vi "getConstants.vi"(0 "niDAQmxAO.lvclass in":refnum<class "niDAQmxAO.lvclass">, 1 "error in (no error)":errorcluster) -> (2 "niDAQmxAO.lvclass out":refnum<class "niDAQmxAO.lvclass">, 3 "Constants":T1={"Configuration Type"={"Differential"=10106, "Pseudodifferential"=12529, "RSE"=10083.0}, "Voltage Type"={"Voltage"="Voltage", "Current"="Current", "Standard Function "={"Sine"="Sine", "Square"="Square", "Triangle"="Triangle"}}}, 4 "error out":errorcluster)   [LabVIEW 2011, in "Hardware.lvlib" / "Channels.lvlib" / "niDAQmxAO.lvclass"]
uses:
  niDAQmxAO.lvclass
  niDAQmxAO.lvclass/niDAQmxAO.ctl
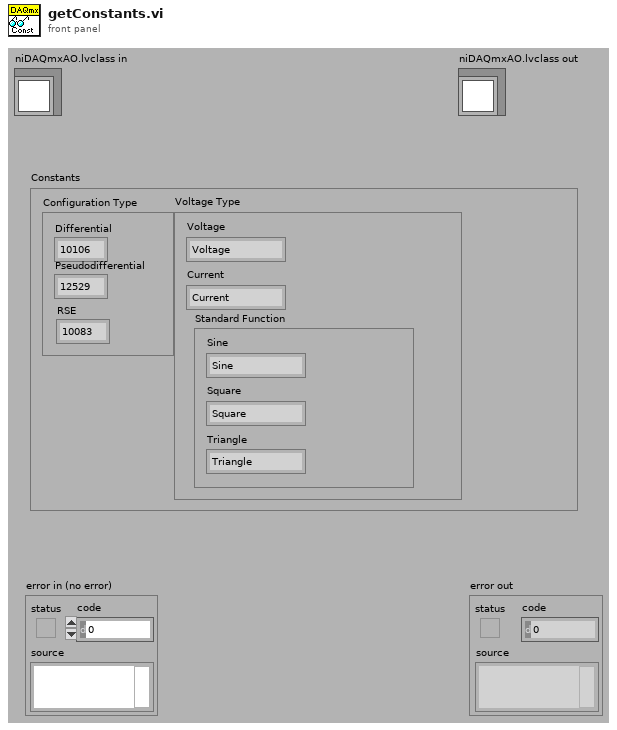
[diagram p1: front panel]
types:
  T1 = cluster{"Configuration Type":cluster{"Differential":i16, "Pseudodifferential":i16, "RSE":dbl}, "Voltage Type":cluster{"Voltage":string, "Current":string, "Standard Function ":cluster{"Sine":string, "Square":string, "Triangle":string}}}
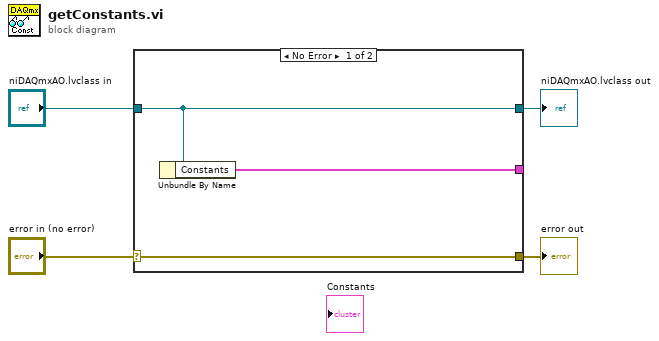
[diagram p0: block diagram]
diagram:
  n1 = case shown="No Error" "error in (no error)" {
    selector: "error in (no error)" -> [w7 w8]
    tunnel: [w7 w8] -> w3
    tunnel: [w6 w9] -> w1
    tunnel: "niDAQmxAO.lvclass in" -> [w6 w9]
    tunnel: [w5 _] -> _
    frame No Error {
      n2 = Unbundle By Name(w6) -> ("Constants"=w5:T1)
    }
    frame Error {
    }
  }
  "error out" <- w3
  "niDAQmxAO.lvclass out" <- w1
